vi "sub_log_basic.vi"(8 "error in":errorcluster, 10 "desc":string, 11 "Title":string) -> (0 "error out":errorcluster)   [LabVIEW 2021]
uses:
  logfile-name.vi
panel:
  out "추가된 경로":path
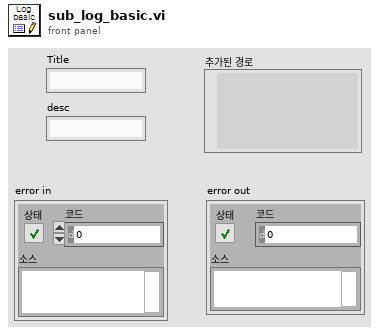
[diagram p1: front panel]
types:
  T1 = enum16{"open", "replace", "create", "open or create", "replace or create", "replace or create with confirmation"}
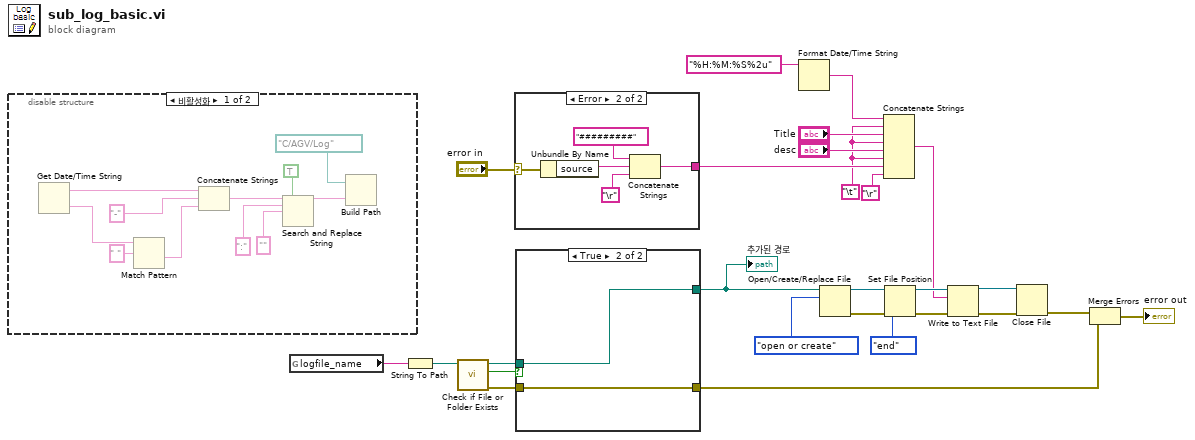
[diagram p0: block diagram]
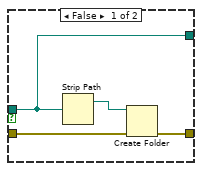
[diagram p4: hidden frame]
diagram:
  w20 = "\t"
  n1 = disable-structure shown="비활성화" {
    frame Disabled {
      n2 = Get Date/Time String() -> (date string=w29:string, time string=w35:string)  [unwired: 3 in]
      n3 = Match Pattern(string=w35, regular expression=" " ("정규식")) -> (after substring=w34:string)  [unwired: 1 in, 3 out]
      n4 = Concatenate Strings(w29, "-" ("정규식"), w34) -> (w30:string)
      n5 = Search and Replace String(replace all?=TRUE ("모두 대체? (거짓)"), input string=w30, search string=":" ("검색 문자열"), replace string="" ("대체 문자열(\"\")")) -> (result string=w27:string)  [unwired: 4 in, 3 out]
      n6 = Build Path(base path=path "C:/AGV/Log" ("베이스 경로"), name or relative path=w27) -> ()  [unwired: 1 out]
    }
    frame Enabled {
    }
  }
  n7 = global read "logfile-name.vi" "logfile_name"() -> (w3:string)
  n8 = String To Path(string=w3) -> (path=w2:path)
  n9 = call <vilib>:"Check if File or Folder Exists.vi"("path"=w2) -> ("error out"=w7:errorcluster, "file or folder exists?"=w8:bool, "dup path"=w26:path)  [unwired: 8 in]
  n10 = case shown="Error" "error in" {
    selector: "error in" -> [_ w42]
    tunnel: [_ w38] -> w21
    frame No Error {
    }
    frame Error {
      n11 = Unbundle By Name(w42) -> ("source"=w40:string)
      n12 = Concatenate Strings("#########" ("문자열"), w40, "\r") -> (w38:string)
    }
  }
  n13 = case shown="True" w8 {
    tunnel: w26 -> [w44 w48]
    tunnel: [w44 w48] -> w1
    tunnel: w7 -> [w46 w47]
    tunnel: [w45 w47] -> w5
    frame False {
      n14 = Strip Path(path=w44) -> (stripped path=w43:path)  [unwired: 1 out]
      n15 = Create Folder(path (use dialog)=w43, error in=w46) -> (error out=w45:errorcluster)  [unwired: 1 in, 2 out]
    }
    frame True {
    }
  }
  "추가된 경로" <- w1
  n16 = Format Date/Time String(time format string (%c)="%H:%M:%S%2u" ("시간 포맷 문자열 (%c)")) -> (date/time string=w24:string)  [unwired: 2 in]
  n17 = Open/Create/Replace File(file path (use dialog)=w1, operation (0:open)=T1."open or create" ("동작(0:open)")) -> (refnum out=w17:refnum<file>, error out=w16:errorcluster)  [unwired: 4 in, 1 out]
  n18 = Concatenate Strings(w24, w20, "Title", w20, "desc", w20, w21, "\r") -> (w10:string)
  n19 = Set File Position(refnum=w17, from (0:start)=enum16{"start", "end", "current"}."end" ("위치(0:start)"), error in=w16) -> (refnum out=w13:refnum<file>, error out=w14:errorcluster)  [unwired: 1 in]
  n20 = Write to Text File(file (use dialog)=w13, text=w10, error in=w14) -> (refnum out=w11:refnum<file>, error out=w12:errorcluster)  [unwired: 1 in, 1 out]
  n21 = Close File(refnum=w11, error in=w12) -> (error out=w6:errorcluster)  [unwired: 1 out]
  n22 = Merge Errors(w6, w5) -> (→"error out":errorcluster)
